vi "reset image texture.vi"(8 "error in (no error)":errorcluster, 10 "Scene:New Object":refnum<vi>, 11 "Array":string[][](array[string])) -> (0 "error out":errorcluster, 3 "Scene.Object Out":refnum<vi>)   [LabVIEW 2019]
uses:
  <vilib>/picture/3D Picture Control/NI_3D Picture Control.lvlib
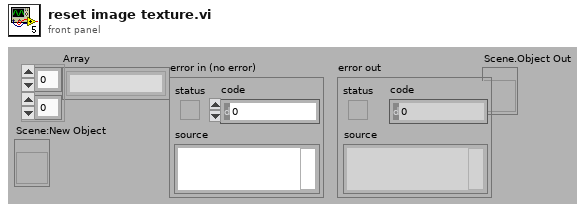
[diagram p1: front panel]
types:
  T1 = typedef "imagedata.ctl" = cluster{"image type":i32, "image depth":i32, "image":u8[], "mask":u8[], "colors":u32[], "Rectangle":cluster{"left":i16, "top":i16, "right":i16, "bottom":i16}}
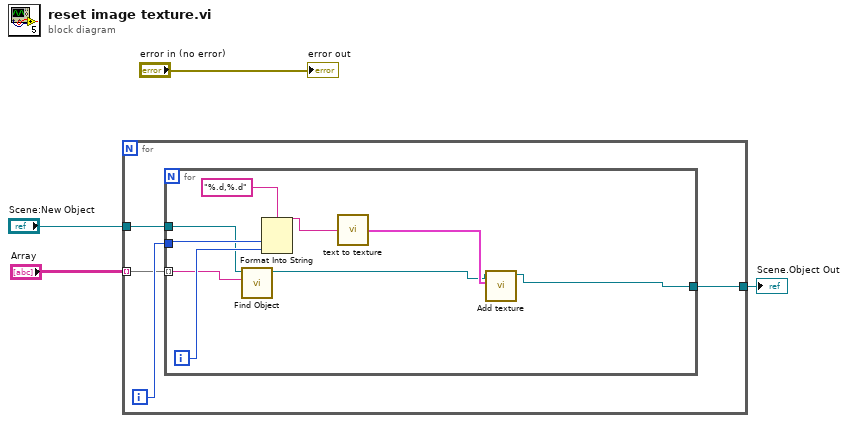
[diagram p0: block diagram]
diagram:
  n1 = for {
    tunnel: "Array" -> [w7] mode=indexing
    tunnel: [w6] -> w3
    tunnel: "Scene:New Object" -> [w5]
    i -> [w8]
    n2 = for {
      tunnel: w8 -> [w14]
      tunnel: w7 -> [w12] mode=indexing
      tunnel: [w10] -> w6
      tunnel: w5 -> [w11]
      i -> [w15]
      n3 = call <vilib>:"Find Object.vi"("Object Name"=w12, "Scene Refnum"=w11) -> ("Object Refnum"=w9:refnum<vi>)  [unwired: 8 in, 1 out]
      n4 = Format Into String(format string="%.d,%.d", w14, w15) -> (resulting string=w13:string)  [unwired: 2 in, 1 out]
      n5 = call "text to texture.vi"("String"=w13) -> ("image data"=w17:T1)
      n6 = call "Add texture.vi"("Image"=w17, "Scene.Object In"=w9) -> ("Scene.Object Out"=w10:refnum<vi>)  [unwired: 9 in]
    }
  }
  "Scene.Object Out" <- w3
  "error out" <- "error in (no error)"
